vi "loadSummaryNew.vi"(9 "machine":string, 11 "path":path=path "C:/temp/summary") -> (0 "error out":errorcluster)   [LabVIEW 2012]
uses:
  <vilib>/addons/database/Connection.llb/DB Tools Open Connec (Path).vi
  <vilib>/addons/database/NI_Database_API.lvlib
panel:
  out "trimmed string":string
  out "concatenated string 2":string
  in  "input cluster 2":T1
  out "concatenated string":string
  out "filenames":string[](array[string])
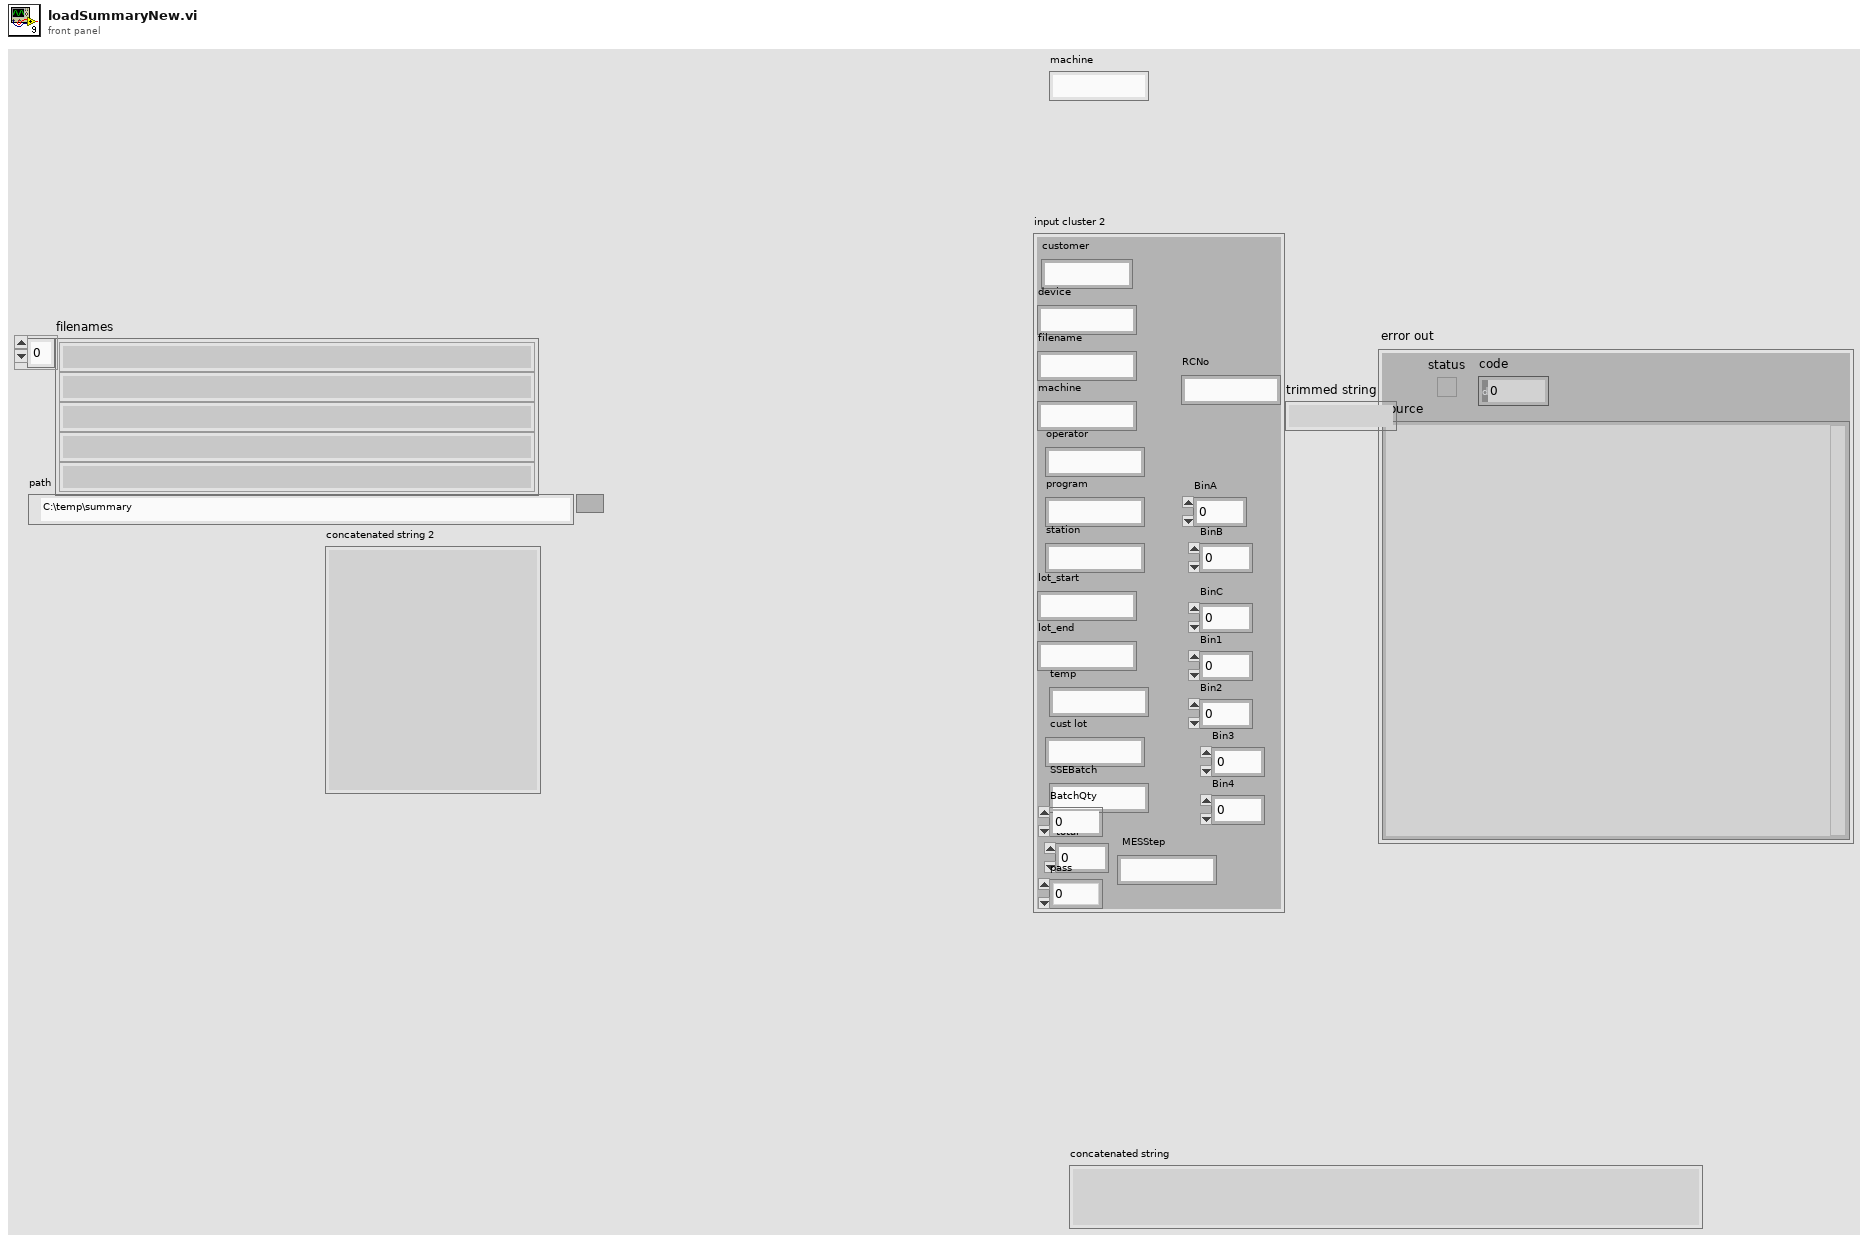
[diagram p1: front panel]
types:
  T1 = cluster{"customer":string, "device":string, "filename":string, "RCNo":string, "machine":string, "operator":string, "program":string, "station":string, "lot_start":string, "lot_end":string, "temp":string, "cust lot":string, "SSEBatch":string, "BatchQty":dbl, "total":dbl, "pass":dbl, "BinA":dbl, "BinB":dbl, "BinC":dbl, "Bin1":dbl, "Bin2":dbl, "Bin3":dbl, "Bin4":dbl, "MESStep":string}
  T2 = typedef "NI_Database_API.lvlib/Conn ObjectReference.ctl" = refnum<k1>
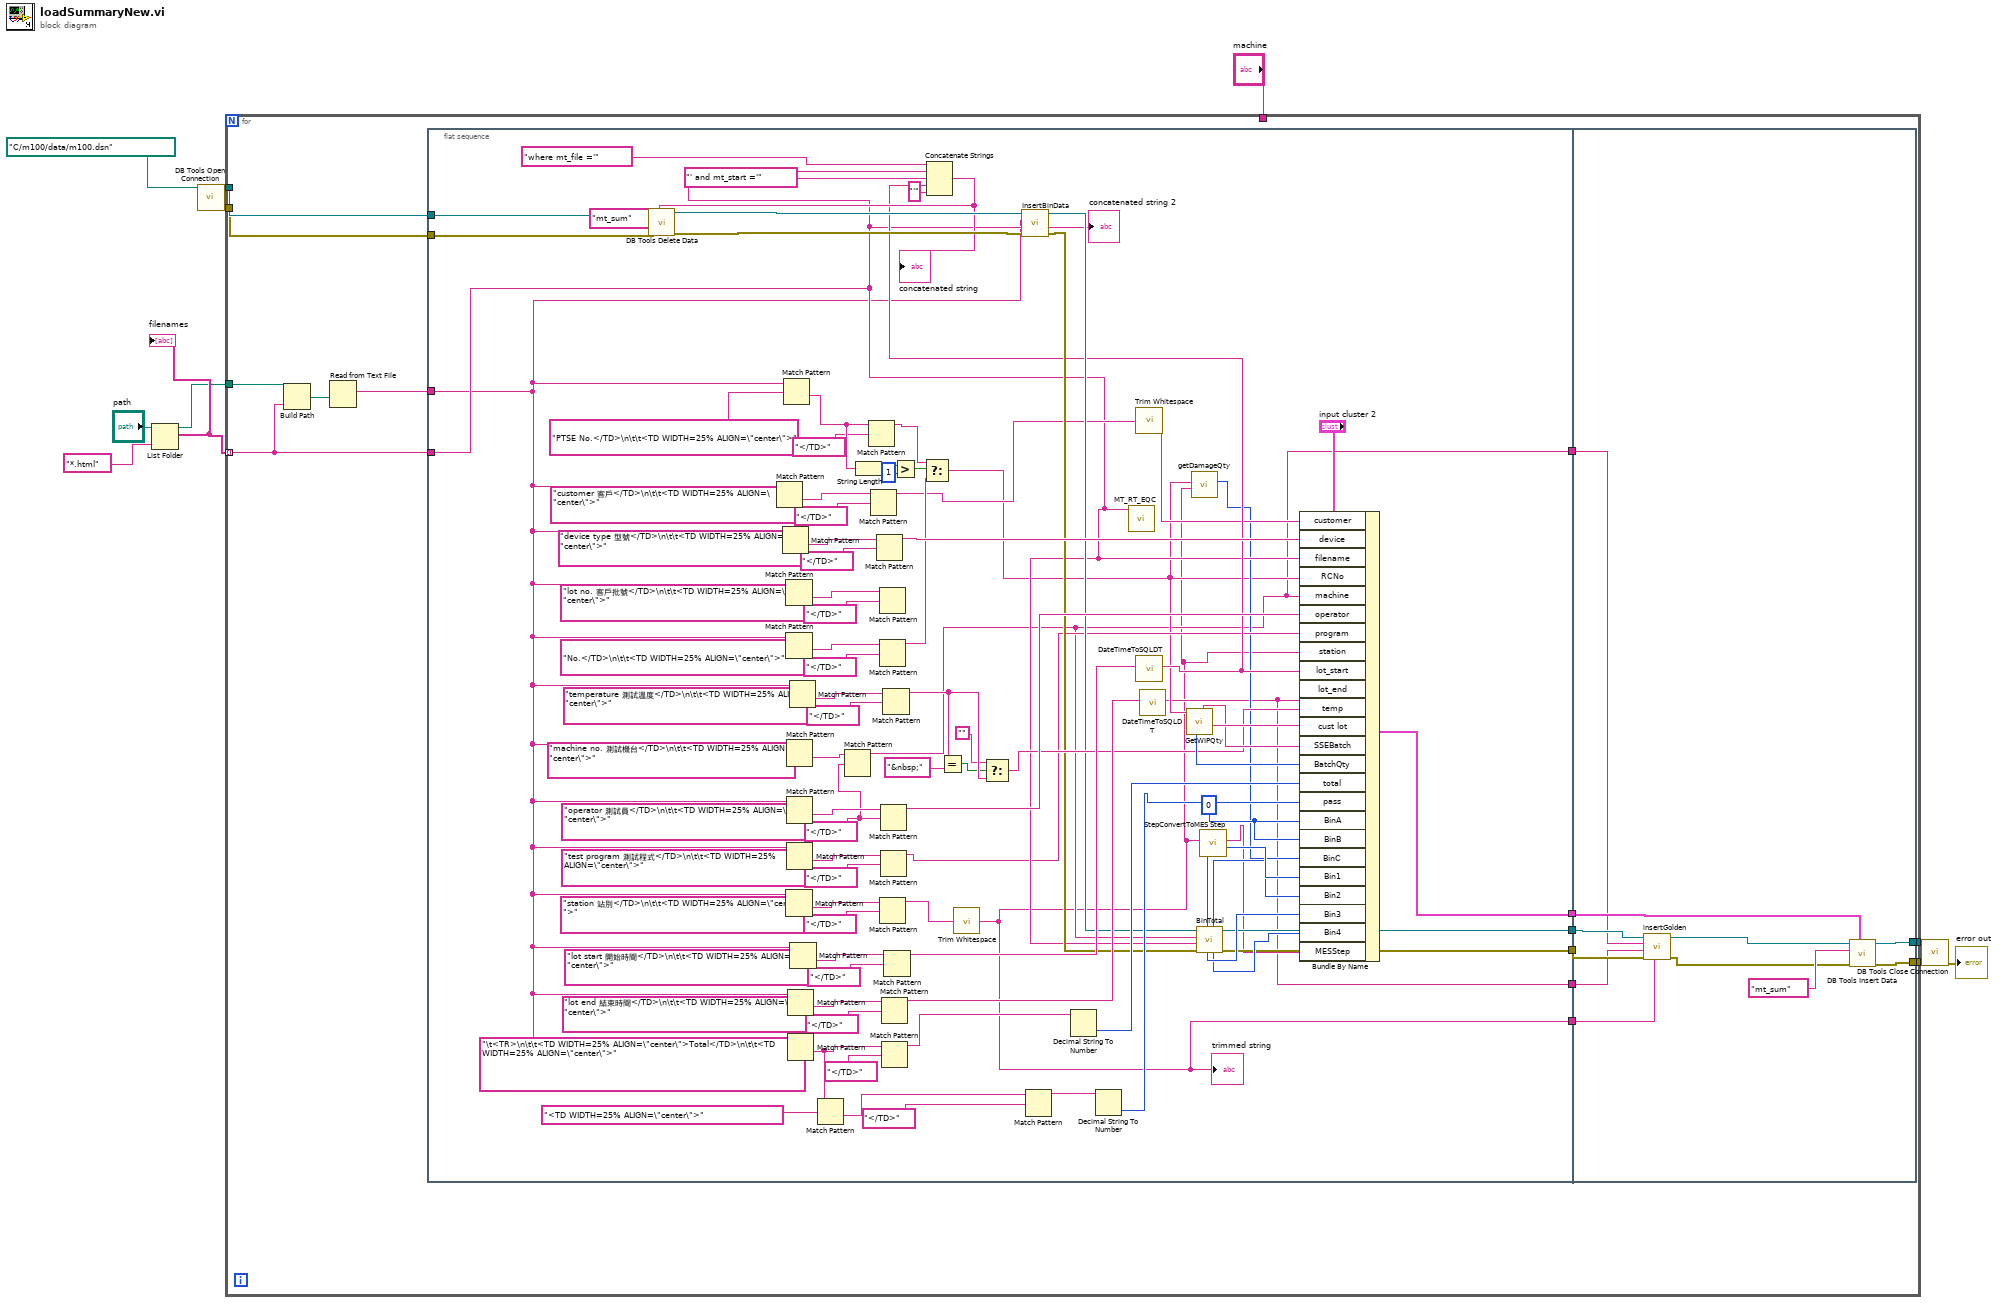
[diagram p0: block diagram]
diagram:
  n1 = List Folder(path="path", pattern="*.html") -> (path out=w9:path, filenames=w10:string[])  [unwired: 2 in, 2 out]
  "filenames" <- w10
  n2 = call-poly <vilib>:"DB Tools Open Connection.vi"("connection information"=path "C:/m100/data/m100.dsn") -> ("error out"=w5:errorcluster, "connection reference"=w6:T2)  [unwired: 7 in]
  n3 = for {
    tunnel: w10 -> [w15] mode=indexing
    tunnel: w9 -> [w24]
    tunnel: w6 -> [w23]
    tunnel: w5 -> [w22]
    tunnel: "machine" -> [_]
    tunnel: [w18] -> w2
    tunnel: [w17] -> w1
    n4 = Build Path(base path=w24, name or relative path=w15) -> (appended path=w25:path)
    n5 = Read from Text File(file (use dialog)=w25) -> (text=w21:string)  [unwired: 3 in, 3 out]
    n6 = flat-sequence {
      tunnel: w23 -> [w44]
      tunnel: w22 -> [w43]
      tunnel: w21 -> [w31]
      tunnel: [w51] -> w20
      tunnel: [w50] -> w19
      tunnel: [w38] -> w16
      tunnel: w15 -> [w34]
      tunnel: [w28] -> w14
      tunnel: [w27] -> w13
      tunnel: [w26] -> w12
      tunnel: w20 -> [w127]
      tunnel: w19 -> [w128]
      tunnel: [w131] -> w18
      tunnel: [w130] -> w17
      tunnel: w16 -> [w132]
      tunnel: w14 -> [w124]
      tunnel: w13 -> [w123]
      tunnel: w12 -> [w122]
      frame #0 {
        w49 = 0
        w58 = "</TD>" ("regular expression")
        n7 = Match Pattern(string=w31, regular expression="customer 客戶</TD>\n\t\t<TD WIDTH=25% ALIGN=\"center\">") -> (after substring=w120:string)  [unwired: 1 in, 3 out]
        n8 = Match Pattern(string=w31, regular expression="device type 型號</TD>\n\t\t<TD WIDTH=25% ALIGN=\"center\">") -> (after substring=w117:string)  [unwired: 1 in, 3 out]
        n9 = Match Pattern(string=w31, regular expression="PTSE No.</TD>\n\t\t<TD WIDTH=25% ALIGN=\"center\">") -> (after substring=w80:string)  [unwired: 1 in, 3 out]
        n10 = Match Pattern(string=w31, regular expression="lot no. 客戶批號</TD>\n\t\t<TD WIDTH=25% ALIGN=\"center\">") -> (after substring=w114:string)  [unwired: 1 in, 3 out]
        n11 = Match Pattern(string=w31, regular expression="No.</TD>\n\t\t<TD WIDTH=25% ALIGN=\"center\">") -> (after substring=w111:string)  [unwired: 1 in, 3 out]
        n12 = Match Pattern(string=w31, regular expression="station 站別</TD>\n\t\t<TD WIDTH=25% ALIGN=\"center\">") -> (after substring=w100:string)  [unwired: 1 in, 3 out]
        n13 = Match Pattern(string=w31, regular expression="machine no. 測試機台</TD>\n\t\t<TD WIDTH=25% ALIGN=\"center\">") -> (after substring=w59:string)  [unwired: 1 in, 3 out]
        n14 = Match Pattern(string=w31, regular expression="operator 測試員</TD>\n\t\t<TD WIDTH=25% ALIGN=\"center\">") -> (after substring=w105:string)  [unwired: 1 in, 3 out]
        n15 = Match Pattern(string=w31, regular expression="test program 測試程式</TD>\n\t\t<TD WIDTH=25% ALIGN=\"center\">") -> (after substring=w103:string)  [unwired: 1 in, 3 out]
        n16 = Match Pattern(string=w31, regular expression="lot end 結束時間</TD>\n\t\t<TD WIDTH=25% ALIGN=\"center\">") -> (after substring=w94:string)  [unwired: 1 in, 3 out]
        n17 = Match Pattern(string=w31, regular expression="\t<TR>\n\t\t<TD WIDTH=25% ALIGN=\"center\">Total</TD>\n\t\t<TD WIDTH=25% ALIGN=\"center\">") -> (after substring=w90:string)  [unwired: 1 in, 3 out]
        n18 = Match Pattern(string=w31, regular expression="temperature 測試溫度</TD>\n\t\t<TD WIDTH=25% ALIGN=\"center\">") -> (after substring=w108:string)  [unwired: 1 in, 3 out]
        n19 = Match Pattern(string=w31, regular expression="lot start 開始時間</TD>\n\t\t<TD WIDTH=25% ALIGN=\"center\">") -> (after substring=w97:string)  [unwired: 1 in, 3 out]
        n20 = Match Pattern(string=w90, regular expression="<TD WIDTH=25% ALIGN=\"center\">") -> (after substring=w87:string)  [unwired: 1 in, 3 out]
        n21 = Match Pattern(string=w59, regular expression=w58) -> (before substring=w28:string)  [unwired: 1 in, 3 out]
        n22 = String Length(string=w80) -> (length=w78:i32)
        n23 = Match Pattern(string=w80, regular expression="</TD>") -> (before substring=w76:string)  [unwired: 1 in, 3 out]
        n24 = Match Pattern(string=w120, regular expression="</TD>") -> (before substring=w37:string)  [unwired: 1 in, 3 out]
        n25 = Match Pattern(string=w117, regular expression="</TD>") -> (before substring=w84:string)  [unwired: 1 in, 3 out]
        n26 = Match Pattern(string=w114, regular expression="</TD>") -> ()  [unwired: 1 in, 4 out]
        n27 = Match Pattern(string=w111, regular expression="</TD>") -> (before substring=w75:string)  [unwired: 1 in, 3 out]
        n28 = Match Pattern(string=w100, regular expression="</TD>") -> (before substring=w35:string)  [unwired: 1 in, 3 out]
        n29 = Match Pattern(string=w105, regular expression=w58) -> (before substring=w83:string)  [unwired: 1 in, 3 out]
        n30 = Match Pattern(string=w103, regular expression="</TD>") -> (before substring=w33:string)  [unwired: 1 in, 3 out]
        n31 = Match Pattern(string=w94, regular expression="</TD>") -> (before substring=w73:string)  [unwired: 1 in, 3 out]
        n32 = Match Pattern(string=w90, regular expression="</TD>") -> (before substring=w86:string)  [unwired: 1 in, 3 out]
        n33 = Match Pattern(string=w108, regular expression="</TD>") -> (before substring=w62:string)  [unwired: 1 in, 3 out]
        n34 = Match Pattern(string=w97, regular expression="</TD>") -> (before substring=w74:string)  [unwired: 1 in, 3 out]
        n35 = Greater?(x=w78, y=1) -> (0:w79:bool)
        n36 = Select(t=w76, s=w79, f=w75) -> (s? t:f=w29:string)
        n37 = Equal?(x=w62, y="&nbsp;") -> (x = y?=w61:bool)
        n38 = call <vilib>:"Trim Whitespace.vi"("string"=w35) -> ("trimmed string"=w26:string)  [unwired: 1 in]
        "trimmed string" <- w26
        n39 = Select(t="", s=w61, f=w62) -> (s? t:f=w63:string)
        n40 = Match Pattern(string=w87, regular expression="</TD>") -> (before substring=w82:string)  [unwired: 1 in, 3 out]
        n41 = Decimal String To Number(string=w86) -> (number=w70:i32)  [unwired: 2 in, 1 out]
        n42 = Decimal String To Number(string=w82) -> (number=w71:i32)  [unwired: 2 in, 1 out]
        n43 = call "MT_RT_EQC.vi"("input string"=w34) -> ()  [unwired: 6 in, 5 out]
        n44 = call <vilib>:"Trim Whitespace.vi"("string"=w37) -> ("trimmed string"=w36:string)  [unwired: 1 in]
        n45 = call "DateTimeToSQLDT.vi"("DateTimeString"=w74) -> ("SQLDateTime"=w40:string)  [unwired: 10 in]
        n46 = Concatenate Strings("where mt_file ='" ("SQL query"), w34, "' and mt_start ='" ("string"), w40, "'" ("string")) -> (w41:string)
        "concatenated string" <- w41
        n47 = call <vilib>:"DB Tools Delete Data.vi"("condition"=w41, "error in (no error)"=w43, "table"="mt_sum", "connection reference"=w44) -> ("error out"=w45:errorcluster, "connection reference out"=w46:T2)  [unwired: 6 in]
        n48 = call "InsertBinData.vi"("error in (no error)"=w45, "FileName"=w34, "string"=w31, "connection reference"=w46) -> ("error out"=w53:errorcluster, "concatenated string"=→"concatenated string 2":string, "connection reference out"=w52:T2)  [unwired: 5 in]
        n49 = call "DateTimeToSQLDT.vi"("DateTimeString"=w73) -> ("SQLDateTime"=w27:string)  [unwired: 10 in]
        n50 = call "GetWIPQty.vi"("Lotno"=w29) -> ("lotno"=w72:string, "SSEBATCH"=w68:string, "BATCHQTY"=w69:i32)  [unwired: 2 in, 6 out]
        n51 = call "getDamageQty.vi"("Step"=w26, "RCNo"=w29) -> ("Damage"=w32:i32)  [unwired: 9 in]
        n52 = call "BinTotal.vi"("error out 2"=w53, "fileName"=w34, "machine"=w28, "connection reference"=w52) -> ("error out"=w50:errorcluster, "connection reference 2"=w51:T2, "bin4"=w54:i32, "bin2"=w56:i32, "bin3"=w55:i32, "bin1"=w57:i32)  [unwired: 2 in]
        n53 = call "StepConvertToMES Step.vi"("Step"=w26) -> ("MES Step"=w39:string)  [unwired: 10 in]
        n54 = Bundle By Name(cluster="input cluster 2", "customer"=w36, "device"=w84, "filename"=w34, "RCNo"=w29, "machine"=w28, "operator"=w83, "program"=w33, "station"=w26, "lot_start"=w40, "lot_end"=w27, "temp"=w63, "cust lot"=w72, "SSEBatch"=w68, "BatchQty"=w69, "total"=w70, "pass"=w71, "BinA"=w49, "BinB"=w49, "BinC"=w32, "Bin1"=w57, "Bin2"=w56, "Bin3"=w55, "Bin4"=w54, "MESStep"=w39) -> (w38:T1)
      }
      frame #1 {
        n55 = call "insertGolden.vi"("Station"=w122, "error in (no error)"=w128, "trans_time"=w123, "machine"=w124, "connection reference"=w127) -> ("error out"=w126:errorcluster, "connection reference 2"=w125:T2)  [unwired: 5 in]
        n56 = call <vilib>:"DB Tools Insert Data.vi"("data"=w132, "error in (no error)"=w126, "table"="mt_sum", "connection reference"=w125) -> ("error out"=w130:errorcluster, "connection reference out"=w131:T2)  [unwired: 6 in]
      }
    }
  }
  n57 = call <vilib>:"DB Tools Close Connection.vi"("error in (no error)"=w1, "connection reference"=w2) -> ("error out"=→"error out":errorcluster)  [unwired: 5 in]
